vi "Dynamics (SubVI).vi"   [LabVIEW 2018]
uses:
  cpp_dll/dynamics.dll
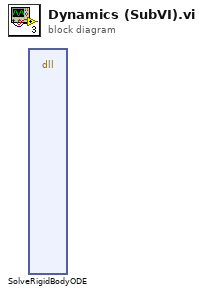
[diagram p0: block diagram]
diagram:
  n1 = dll-call lib="D:/ADCS_lABVIEW/cpp_dll/dynamics.dll" fn="SolveRigidBodyODE"() -> ()  [unwired: 54 in, 2 out]
